vi "test Parsed XML to System Definition.vi"(8 "error in":errorcluster, 11 "TestCase in":refnum<class "Scripting.lvclass">) -> (0 "error out":errorcluster, 3 "TestCase out":refnum<class "Scripting.lvclass">)   [LabVIEW 2020, in "Scripting.lvclass"]
uses:
  Scripting.lvclass
  Shared/VS Channels Definition for All Labels on Hardware Channel.ctl
  Shared/Direction.ctl
  Shared/VS Channels Definition for Label.ctl
  Shared/VS Channel Definition for Parameter.ctl
  Shared/Parameter Definition.ctl
  <vilib>/NI/NI VeriStand Encoding and Decoding/Encoding.ctl
  Shared/Transfer Type.ctl
  Scripting.lvclass/Scripting.ctl
  <vilib>/addons/_JKI Toolkits/VI Tester/TestCase.llb/TestCase.lvclass
  Scripting/AIM/AIM ARINC 429 Scripting.lvlib
  niveristand-custom-device-testing-tools/VeriStandTestUtilities/VeriStandTestUtilities.lvlib
  Scripting/ARINC 429/ARINC 429 Scripting.lvlib
  <vilib>/NI/NI VeriStand Encoding and Decoding/Encoding and Decoding.lvlib
  C:/Program Files (x86)/National Instruments/LabVIEW 2020/vi.lib/addons/_JKI Toolkits/VI Tester/TestCase.llb/TestCase.lvclass
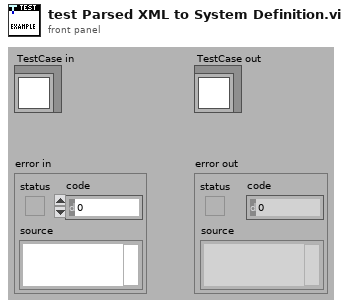
[diagram p1: front panel]
types:
  T1 = typedef "VS Channels Definition for All Labels on Hardware Channel.ctl" = cluster{"hardware channel":i32, "direction":T2, "labels":T3[]}
  T2 = typedef "Direction.ctl" = enum16{"Rx", "Tx"}
  T3 = typedef "VS Channels Definition for Label.ctl" = cluster{"label (Dec)":u32, "parameters":T4[], "SDI value":u8, "SDI enabled":bool, "transfer type":T7, "create timestamp":bool}
  T4 = typedef "VS Channel Definition for Parameter.ctl" = cluster{"name":string, "default value":dbl, "unit":string, "Parameter":T5}
  T5 = typedef "Parameter Definition.ctl" = cluster{"start index":i32, "size":i32, "encoding":T6, "signed":bool, "scale multiplier":dbl, "scale offset":dbl}
  T6 = typedef "Encoding and Decoding.lvlib/Encoding.ctl" = enum16{"BNR", "BCD", "Discrete"}
  T7 = typedef "Transfer Type.ctl" = enum16{"Scheduled", "Acyclic", "Block", "Strobe"}
  T8 = typedef "Custom Device API.lvlib/Custom Device Item Ref.ctl" = u64
  T9 = typedef "Label Properties.ctl" = cluster{"label (Dec)":T10, "SDI value":u8, "SDI enabled":bool}
  T10 = typedef "Label.ctl" = u8
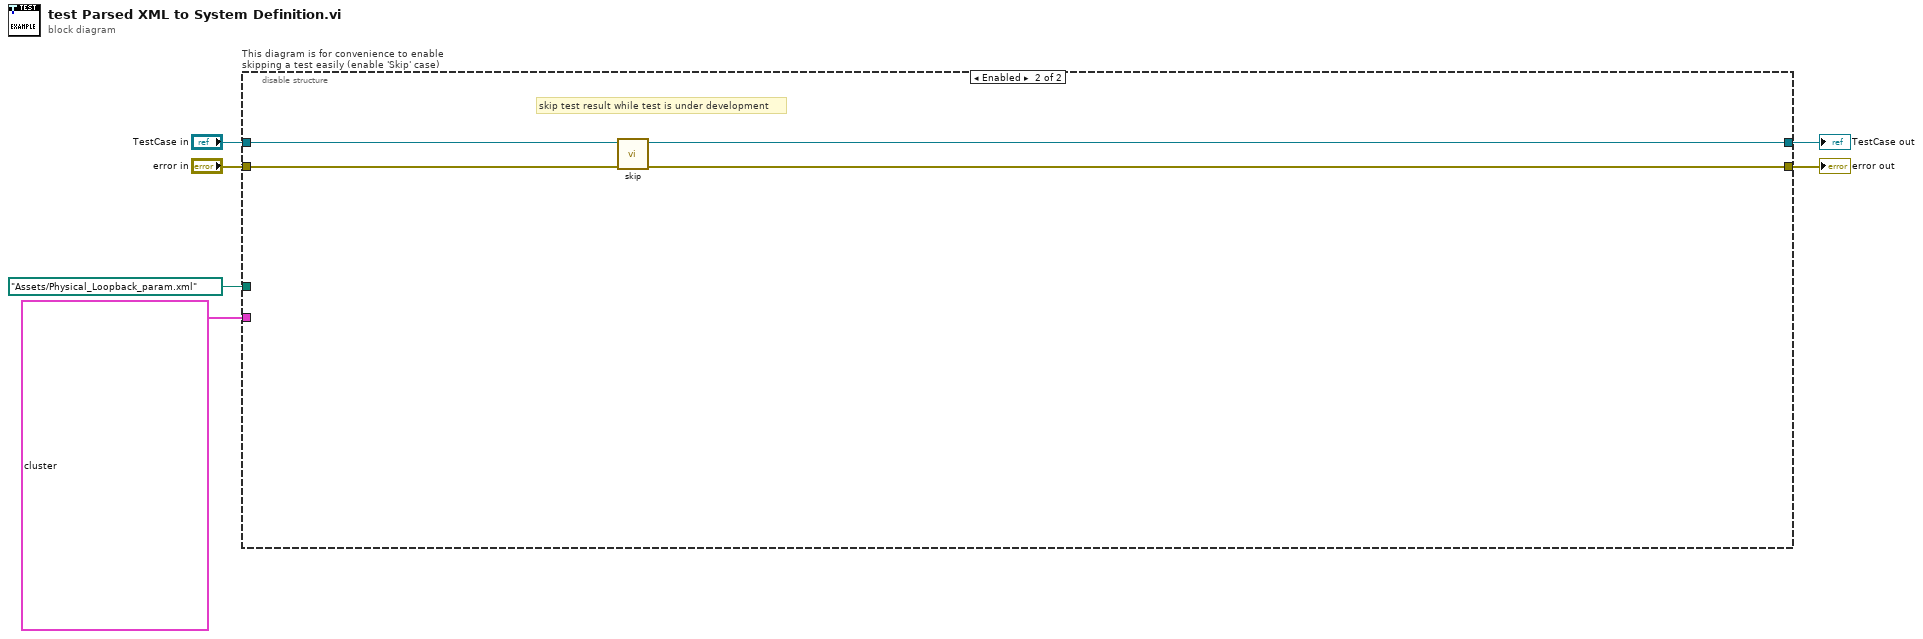
[diagram p0: block diagram]
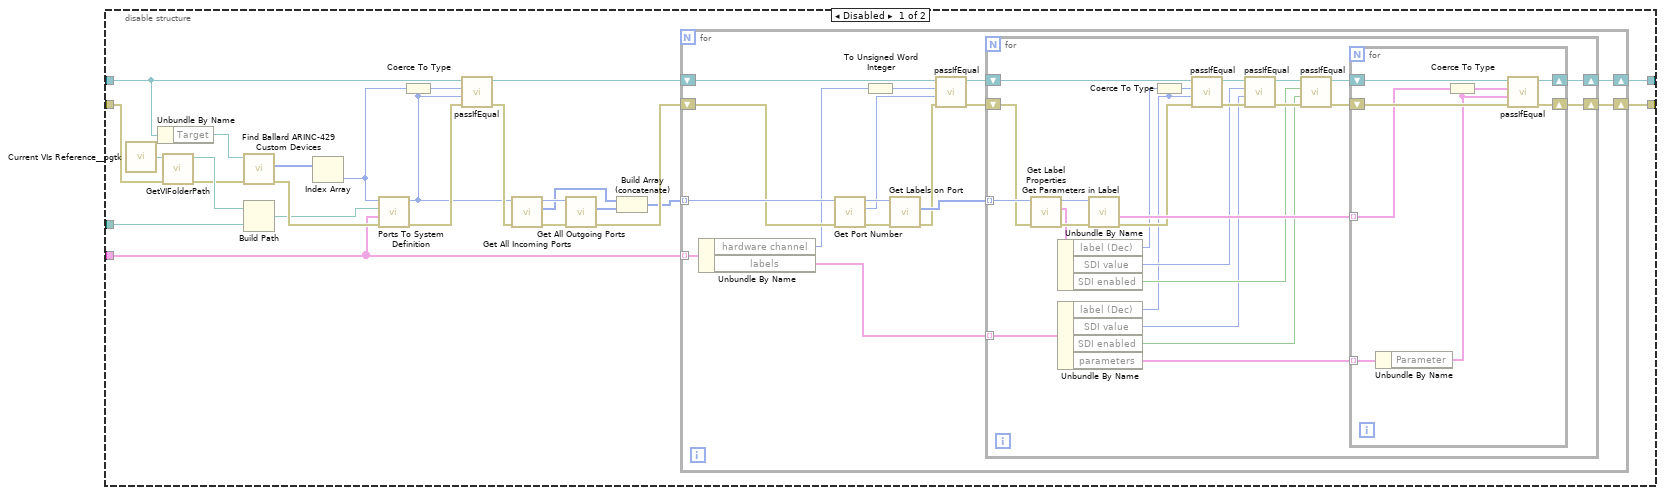
[diagram p2: hidden frame]
diagram:
  n1 = disable-structure "This diagram is for convenience to enable skipping a test easily (enable 'Skip' case)" shown="Enabled" {
    disable-tunnel: "TestCase in" -> [w24 w84]
    disable-tunnel: [w14 w82] -> w3
    disable-tunnel: [w12 w83] -> w5
    disable-tunnel: "error in" -> [w27 w81]
    disable-tunnel: T1[] [{"hardware channel"=0, "direction"=enum."Rx", "labels"=[{"label (Dec)"=134, "parameters"=[{"name"="Altitude_Rx", "default value"=0.0, "unit"="psi", "Parameter"={"start index"=18, "size"=10, "encoding"=enum."BNR", "signed"=TRUE, "scale multiplier"=16.0, "scale offset"=0.0}}, {"name"="SSM", "default value"=0.0, "unit"="", "Parameter"={"start index"=29, "size"=2, "encoding"=enum."BNR", "signed"=FALSE, "scale multiplier"=1.0, "scale offset"=0.0}}], "SDI value"=0, "SDI enabled"=FALSE, "transfer type"=enum."Scheduled", "create timestamp"=FALSE}]}, {"hardware channel"=2, "direction"=enum."Rx", "labels"=[{"label (Dec)"=135, "parameters"=[{"name"="Altitude_Rx", "default value"=0.0, "unit"="ft", "Parameter"={"start index"=10, "size"=19, "encoding"=enum."BCD", "signed"=TRUE, "scale multiplier"=1.0, "scale offset"=0.0}}, {"name"="SSM", "default value"=0.0, "unit"="", "Parameter"={"start index"=29, "size"=2, "encoding"=enum."BNR", "signed"=FALSE, "scale multiplier"=1.0, "scale offset"=0.0}}], "SDI value"=0, "SDI enabled"=FALSE, "transfer type"=enum."Scheduled", "create timestamp"=FALSE}]}, {"hardware channel"=4, "direction"=enum."Rx", "labels"=[{"label (Dec)"=136, "parameters"=[{"name"="Altitude_Rx", "default value"=0.0, "unit"="m", "Parameter"={"start index"=13, "size"=16, "encoding"=enum."BNR", "signed"=TRUE, "scale multiplier"=1.0, "scale offset"=0.0}}, {"name"="valid_Rx", "default value"=0.0, "unit"="", "Parameter"={"start index"=10, "size"=1, "encoding"=enum."Discrete", "signed"=FALSE, "scale multiplier"=1.0, "scale offset"=0.0}}, {"name"="current_Rx", "default value"=0.0, "unit"="", "Parameter"={"start index"=11, "size"=1, "encoding"=enum."Discrete", "signed"=FALSE, "scale multiplier"=1.0, "scale offset"=0.0}}, {"name"="SSM", "default value"=0.0, "unit"="", "Parameter"={"start index"=29, "size"=2, "encoding"=enum."BNR", "signed"=FALSE, "scale multiplier"=1.0, "scale offset"=0.0}}], "SDI value"=0, "SDI enabled"=FALSE, "transfer type"=enum."Scheduled", "create timestamp"=FALSE}]}, {"hardware channel"=17, "direction"=enum."Rx", "labels"=[{"label (Dec)"=134, "parameters"=[{"name"="Altitude_Tx", "default value"=0.0, "unit"="psi", "Parameter"={"start index"=18, "size"=10, "encoding"=enum."BNR", "signed"=TRUE, "scale multiplier"=16.0, "scale offset"=0.0}}], "SDI value"=0, "SDI enabled"=FALSE, "transfer type"=enum."Scheduled", "create timestamp"=FALSE}]}, {"hardware channel"=19, "direction"=enum."Rx", "labels"=[{"label (Dec)"=135, "parameters"=[{"name"="Altitude_Tx", "default value"=0.0, "unit"="ft", "Parameter"={"start index"=10, "size"=19, "encoding"=enum."BCD", "signed"=TRUE, "scale multiplier"=1.0, "scale offset"=0.0}}], "SDI value"=0, "SDI enabled"=FALSE, "transfer type"=enum."Scheduled", "create timestamp"=FALSE}]}, {"hardware channel"=21, "direction"=enum."Rx", "labels"=[{"label (Dec)"=136, "parameters"=[{"name"="Altitude_Tx", "default value"=0.0, "unit"="m", "Parameter"={"start index"=13, "size"=16, "encoding"=enum."BNR", "signed"=TRUE, "scale multiplier"=1.0, "scale offset"=0.0}}, {"name"="valid_Tx", "default value"=0.0, "unit"="", "Parameter"={"start index"=10, "size"=1, "encoding"=enum."Discrete", "signed"=FALSE, "scale multiplier"=1.0, "scale offset"=0.0}}, {"name"="current_Tx", "default value"=0.0, "unit"="", "Parameter"={"start index"=11, "size"=1, "encoding"=enum."Discrete", "signed"=FALSE, "scale multiplier"=1.0, "scale offset"=0.0}}], "SDI value"=0, "SDI enabled"=FALSE, "transfer type"=enum."Scheduled", "create timestamp"=FALSE}]}] ("ports") -> [w8 _]
    disable-tunnel: path "Assets/Physical_Loopback_param.xml" ("Absolute or Relative Path") -> [w25 _]
    frame Disabled {
      n2 = call <userlib>:"Current VIs Reference__ogtk.vi"() -> ("Current VI's reference"=w28:refnum<vi>)  [unwired: 5 in]
      n3 = Unbundle By Name(w24) -> ("Target"=w31:refnum<k24>)
      n4 = call "GetVIFolderPath.vi"("error in (no error)"=w27, "VI Reference in"=w28) -> ("error out"=w26:errorcluster, "VI Folder Path out"=w29:path)  [unwired: 8 in]
      n5 = call "Find Ballard ARINC-429 Custom Devices.vi"("error in"=w26, "target in"=w31) -> ("error out"=w30:errorcluster, "Ballard ARINC 429 custom devices"=w7:u64[])  [unwired: 7 in, 1 out]
      n6 = Build Path(base path=w29, name or relative path=w25) -> (appended path=w9:path)
      n7 = Index Array(array=w7) -> (element=w22:u64)  [unwired: 1 in]
      n8 = call "Ports To System Definition.vi"("error in"=w30, "ports"=w8, "parameter configuration file path"=w9, "custom device ref"=w22) -> ("error out"=w23:errorcluster, "custom device ref out"=w10:T8)  [unwired: 6 in]
      n9 = Coerce To Type(0:w22, 1:w10) -> (2:w11:T8)
      n10 = call-dynamic "passIfEqual.vi"("error in (no error)"=w23, "y"=w10, "x"=w11, "TestCase in"=w24) -> ("error out"=w21:errorcluster, "TestCase out"=w13:refnum<class "Scripting.lvclass">)  [unwired: 6 in]
      n11 = call "Get All Incoming Ports.vi"("error in"=w21, "Ballard ARINC 429 custom device in"=w10) -> ("error out"=w19:errorcluster, "incoming ports"=w16:T8[], "Ballard ARINC 429 custom device out"=w20:T8)  [unwired: 7 in]
      n12 = call "Get All Outgoing Ports.vi"("error in"=w19, "Ballard ARINC 429 custom device in"=w20) -> ("error out"=w18:errorcluster, "outgoing ports"=w17:T8[])  [unwired: 7 in, 1 out]
      n13 = Build Array (concatenate)(w16, w17) -> (w15:T8[])
      n14 = for {
        tunnel: w15 -> [w45] mode=indexing
        tunnel: w8 -> [w47] mode=indexing
        shift-right: [w42] -> w12
        shift-left: w18 -> [w44]
        shift-right: [w33] -> w14
        shift-left: w13 -> [w39]
        n15 = Unbundle By Name(w47) -> ("hardware channel"=w38:i32, "labels"=w40:T3[])
        n16 = call "Get Port Number.vi"("error in"=w44, "port ref in"=w45) -> ("error out"=w43:errorcluster, "port number"=w37:u16, "port ref out"=w46:T8)  [unwired: 6 in, 1 out]
        n17 = To Unsigned Word Integer(number=w38) -> (unsigned 16bit integer=w32:u16)
        n18 = call "Get Labels on Port.vi"("error in"=w43, "port in"=w46) -> ("error out"=w36:errorcluster, "labels"=w41:T8[])  [unwired: 6 in, 2 out]
        n19 = call-dynamic "passIfEqual.vi"("error in (no error)"=w36, "y"=w37, "x"=w32, "TestCase in"=w39) -> ("error out"=w35:errorcluster, "TestCase out"=w34:refnum<class "Scripting.lvclass">)  [unwired: 6 in]
        n20 = for {
          shift-right: [w54] -> w42
          shift-left: w35 -> [w71]
          tunnel: w41 -> [w72] mode=indexing
          tunnel: w40 -> [w68] mode=indexing
          shift-right: [w55] -> w33
          shift-left: w34 -> [w60]
          n21 = call "Get Label Properties.vi"("error in"=w71, "label ref in"=w72) -> ("error out"=w70:errorcluster, "label properties"=w67:T9, "label ref out"=w69:T8)  [unwired: 6 in, 1 out]
          n22 = Unbundle By Name(w67) -> ("label (Dec)"=w49:T10, "SDI value"=w58:u8, "SDI enabled"=w53:bool)
          n23 = Unbundle By Name(w68) -> ("label (Dec)"=w50:u32, "SDI value"=w51:u8, "SDI enabled"=w52:bool, "parameters"=w65:T4[])
          n24 = call "Get Parameters in Label.vi"("error in"=w70, "label in"=w69) -> ("error out"=w59:errorcluster, "parameter definitions"=w66:T5[])  [unwired: 6 in, 2 out]
          n25 = Coerce To Type(0:w49, 1:w50) -> (2:w48:u32)
          n26 = call-dynamic "passIfEqual.vi"("error in (no error)"=w59, "y"=w50, "x"=w48, "TestCase in"=w60) -> ("error out"=w61:errorcluster, "TestCase out"=w62:refnum<class "Scripting.lvclass">)  [unwired: 6 in]
          n27 = call-dynamic "passIfEqual.vi"("error in (no error)"=w61, "y"=w51, "x"=w58, "TestCase in"=w62) -> ("error out"=w64:errorcluster, "TestCase out"=w63:refnum<class "Scripting.lvclass">)  [unwired: 6 in]
          n28 = call-dynamic "passIfEqual.vi"("error in (no error)"=w64, "y"=w52, "x"=w53, "TestCase in"=w63) -> ("error out"=w56:errorcluster, "TestCase out"=w57:refnum<class "Scripting.lvclass">)  [unwired: 6 in]
          n29 = for {
            tunnel: w66 -> [w77] mode=indexing
            tunnel: w65 -> [w80] mode=indexing
            shift-right: [w75] -> w55
            shift-left: w57 -> [w79]
            shift-right: [w76] -> w54
            shift-left: w56 -> [w78]
            n30 = Unbundle By Name(w80) -> ("Parameter"=w73:T5)
            n31 = Coerce To Type(0:w77, 1:w73) -> (2:w74:T5)
            n32 = call-dynamic "passIfEqual.vi"("error in (no error)"=w78, "y"=w73, "x"=w74, "TestCase in"=w79) -> ("error out"=w76:errorcluster, "TestCase out"=w75:refnum<class "Scripting.lvclass">)  [unwired: 6 in]
          }
        }
      }
    }
    frame Enabled {
      # "skip test result while test is under development"
      n33 = call <vilib>:"skip.vi"("error in (no error)"=w81, "TestCase in"=w84) -> ("error out"=w83:errorcluster, "TestCase out"=w82:refnum<class "Scripting.lvclass">)  [unwired: 8 in]
    }
  }
  "error out" <- w5
  "TestCase out" <- w3
